vi "common_GUI_UpdateAliasList.vi"(8 "error in (no error)":errorcluster, 9 "Controls[]":refnum<vi>[](array[refnum]), 10 "Arguments":string, 11 "SQL Server Info":T2) -> (0 "error out":errorcluster)   [LabVIEW 2013]
uses:
  shared programs/MySQL/typedefs/mysql_authentication.ctl
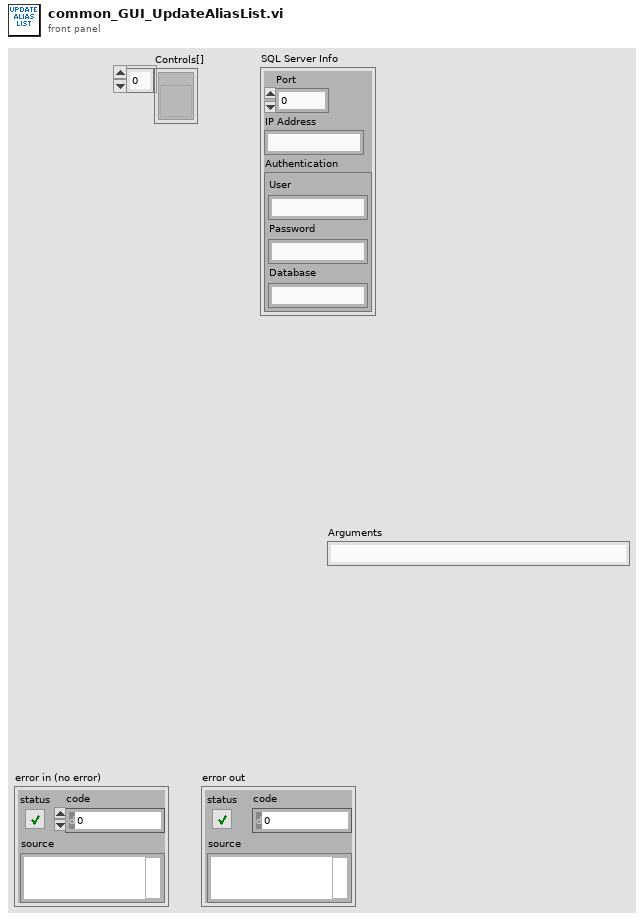
[diagram p1: front panel]
types:
  T1 = typedef "mysql_authentication.ctl" = cluster{"User":string, "Password":string, "Database":string}
  T2 = cluster{"Port":u16, "IP Address":string, "Authentication":T1}
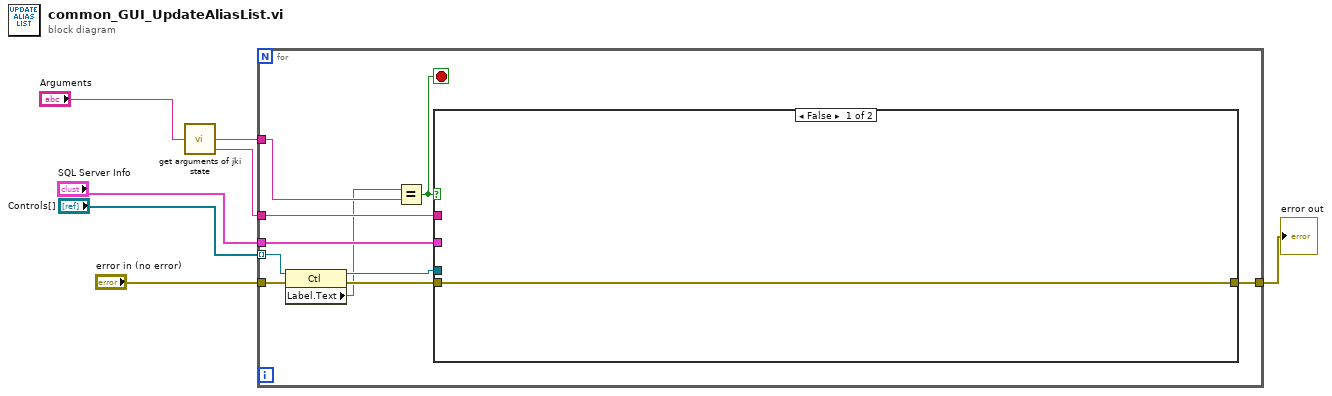
[diagram p0: block diagram]
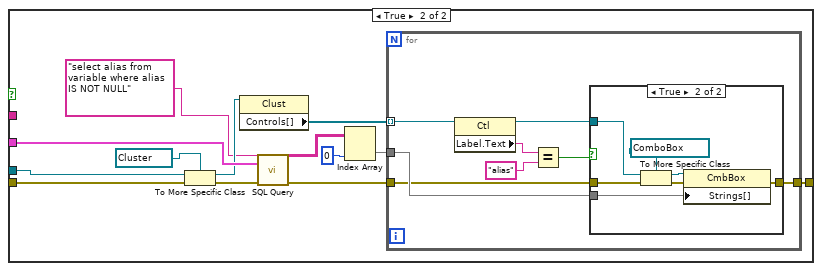
[diagram p2: hidden frame]
diagram:
  n1 = call "get arguments of jki state.vi"("jki arguments"="Arguments") -> ("Arg 1"=w6:string, "Arg 2"=w7:string)  [unwired: 1 out]
  n2 = for {
    tunnel: "Controls[]" -> [w17] mode=indexing
    tunnel: w6 -> [w9]
    tunnel: "error in (no error)" -> [w14]
    tunnel: "SQL Server Info" -> [w13]
    tunnel: [w12] -> w2
    tunnel: w7 -> [w11]
    stop <- w10 stop-if-true
    n3 = property class="Ctl"(reference=w17, error in=w14) -> (reference out=w16:refnum<vi>, error out=w15:errorcluster, "Label.Text"=w8:string)
    n4 = Equal?(x=w8, y=w9) -> (x = y?=w10:bool)
    n5 = case shown="False" w10 {
      tunnel: w16 -> [_ w31]
      tunnel: w15 -> [w18 w30]
      tunnel: w11 -> [_ _]
      tunnel: w13 -> [_ w26]
      tunnel: [w18 w23] -> w12
      frame False {
      }
      frame True {
        n6 = To More Specific Class(target class=refnum<vi> refnum ("Device 2"), reference=w31, error in=w30) -> (specific class reference=w21:refnum<vi>, error out=w25:errorcluster)
        n7 = property class="Clust"(reference=w21) -> ("Controls[]"=w20:refnum<vi>[])  [unwired: 1 in, 2 out]
        n8 = call "SQL Query.vi"("error in (no error)"=w25, "SQL Server Info"=w26, "Query"="select alias from variable where alias IS NOT NULL") -> ("error out"=w24:errorcluster, "data"=w29:string[][])  [unwired: 7 in]
        n9 = Index Array(array=w29, index (col)=0 ("disabled index (col)")) -> (element=w27:string[])  [unwired: 1 in]
        n10 = for {
          tunnel: w27 -> [w39]
          tunnel: w24 -> [w37]
          tunnel: [w38] -> w23
          tunnel: w20 -> [w36] mode=indexing
          n11 = property class="Ctl"(reference=w36) -> (reference out=w34:refnum<vi>, "Label.Text"=w33:string)  [unwired: 1 in, 1 out]
          n12 = Equal?(x=w33, y="alias") -> (x = y?=w32:bool)
          n13 = case shown="True" w32 {
            tunnel: w39 -> [_ w47]
            tunnel: [w40 w46] -> w38
            tunnel: w37 -> [w40 w43]
            tunnel: w34 -> [_ w41]
            frame False {
            }
            frame True {
              n14 = To More Specific Class(target class=refnum<vi> refnum ("Device 2"), reference=w41, error in=w43) -> (specific class reference=w44:refnum<vi>, error out=w42:errorcluster)
              n15 = property class="CmbBox"(reference=w44, error in=w42, "Strings[]"=w47) -> (error out=w46:errorcluster)  [unwired: 1 out]
            }
          }
        }
      }
    }
  }
  "error out" <- w2
